vi "Teleop.vi"(10 "Match Info":T1={"Autonomous Elapsed Seconds"=0.0, "TeleOp Elapsed Seconds"=0.0, "Disabled Elapsed Seconds"=0.0, "Visited Autonomous"=FALSE, "Visited TeleOp"=FALSE, "Visited Disabled"=FALSE, "Autonomous Settings"={"Autonomous Style"=enum."Independent", "VI Refnum"=refnum}}, 11 "Call Context":T2) -> ()   [LabVIEW 2023]
doc: "This VI is called for each TeleOp packet received from the DS where the robot is not disabled. It is often used to read from the joysticks and update I/O or to update setpoints for timed control loops. It should complete and return within 20 milliseconds or it may miss DS packets."
uses:
  <vilib>/Rock Robotics/WPI/DriverStation/WPI_DriverStationDerivedRobotMode.ctl
  <vilib>/Rock Robotics/WPI/DriverStation/WPI_DriverStationMatch Info.ctl
  <vilib>/Rock Robotics/WPI/Utilities/WPI_GetSetVariantRefNum.vi
  <vilib>/Rock Robotics/Network Tables/NT Write Boolean Array.vi
  <vilib>/Rock Robotics/Network Tables/NT Write Numeric Array.vi
  <vilib>/Rock Robotics/Network Tables/NT Write Boolean.vi
  <vilib>/Rock Robotics/Network Tables/NT Read Boolean.vi
  <vilib>/Rock Robotics/Network Tables/NT Read Number.vi
  <vilib>/Rock Robotics/WPI/RobotDrive/WPI_RobotDriveMecanumDrive_Cartesian.vi
panel:
  out "Sample Slider 0":dbl(slide) scale=0.0..5.0
  out "Sample Boolean 1":bool
  out "Sample Boolean 0":bool
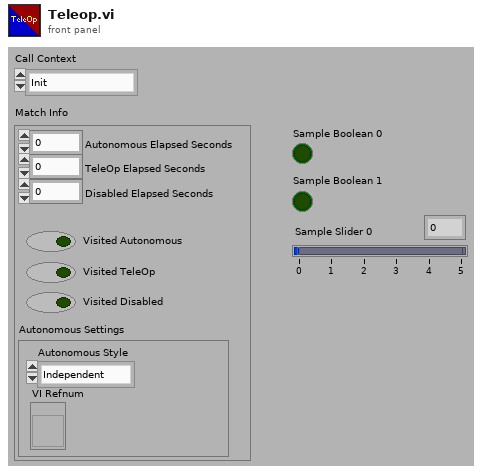
[diagram p1: front panel]
types:
  T1 = typedef "WPI_DriverStationMatch Info.ctl" = cluster{"Autonomous Elapsed Seconds":dbl, "TeleOp Elapsed Seconds":dbl, "Disabled Elapsed Seconds":dbl, "Visited Autonomous":bool, "Visited TeleOp":bool, "Visited Disabled":bool, "Autonomous Settings":cluster{"Autonomous Style":enum16{"Iterative", "Independent"}, "VI Refnum":refnum<vi>}}
  T2 = typedef "WPI_DriverStationDerivedRobotMode.ctl" = enum16{"Init", "Execute", "Stop"}
  T3 = typedef "WPI_MotorControlDeviceRef.ctl" = cluster{"DeviceStatus":errorcluster, "Type":T4, "PWM":cluster{"PWM Channel":T5, "DeadBand":T6}, "CAN":cluster{"Device Number":u8, "SetOutput VI Ref":variant, "GetOutput VI Ref":variant, "Enable VI Ref":variant, "Disable VI Ref":variant, "Data":variant}, "Invert":bool, "DIO PWM":cluster{"PWM \"Enable\" Channel":T5, "DIOChannel":T7, "PWM Rate":dbl}}
  T4 = typedef "WPI_MotorControlType.ctl" = enum16{"PWM", "CAN", "DIO PWM"}
  T5 = typedef "FPGA_DIOPWMChannel.ctl" = enum8{"PWM 0", "PWM 1", "PWM 2", "PWM 3", "PWM 4", "PWM 5", "PWM 6", "PWM 7", "PWM 8", "PWM 9", "PWM MXP 0", "PWM MXP 1", "PWM MXP 2", "PWM MXP 3", "PWM MXP 4", "PWM MXP 5", "PWM MXP 6", "PWM MXP 7", "PWM MXP 8", "PWM MXP 9", "Invalid"}
  T6 = typedef "WPI_PWMDeadband.ctl" = cluster{"Name":string, "maxPositivePwm":i32, "minPositivePwm":i32, "centerPwm":i32, "maxNegativePwm":i32, "minNegativePwm":i32, "angularRange":u16}
  T7 = typedef "FPGA_DIOChannel.ctl" = enum8{"DIO 0", "DIO 1", "DIO 2", "DIO 3", "DIO 4", "DIO 5", "DIO 6", "DIO 7", "DIO 8", "DIO 9", "DIO MXP 0", "DIO MXP 1", "DIO MXP 2", "DIO MXP 3", "DIO MXP 4", "DIO MXP 5", "DIO MXP 6", "DIO MXP 7", "DIO MXP 8", "DIO MXP 9", "DIO MXP 10", "DIO MXP 11", "DIO MXP 12", "DIO MXP 13", "DIO MXP 14", "DIO MXP 15", "SPI Port CS1", "SPI Port CS2", "SPI Port CS3", "SPI Port MISO", "SPI Port MOSI", "Invalid"}
  T8 = typedef "WPI_JoystickDevRef.ctl" = cluster{"Device":T9}
  T9 = typedef "WPI_JoystickDeviceEnum.ctl" = enum16{"USB 0", "USB 1", "USB 2", "USB 3", "USB 4", "USB 5"}
  T10 = typedef "WPI_RobotDriveDevRef.ctl" = cluster{"DevStatus":errorcluster, "Motors[]":T3[], "Square Inputs":bool, "Max Output":dbl}
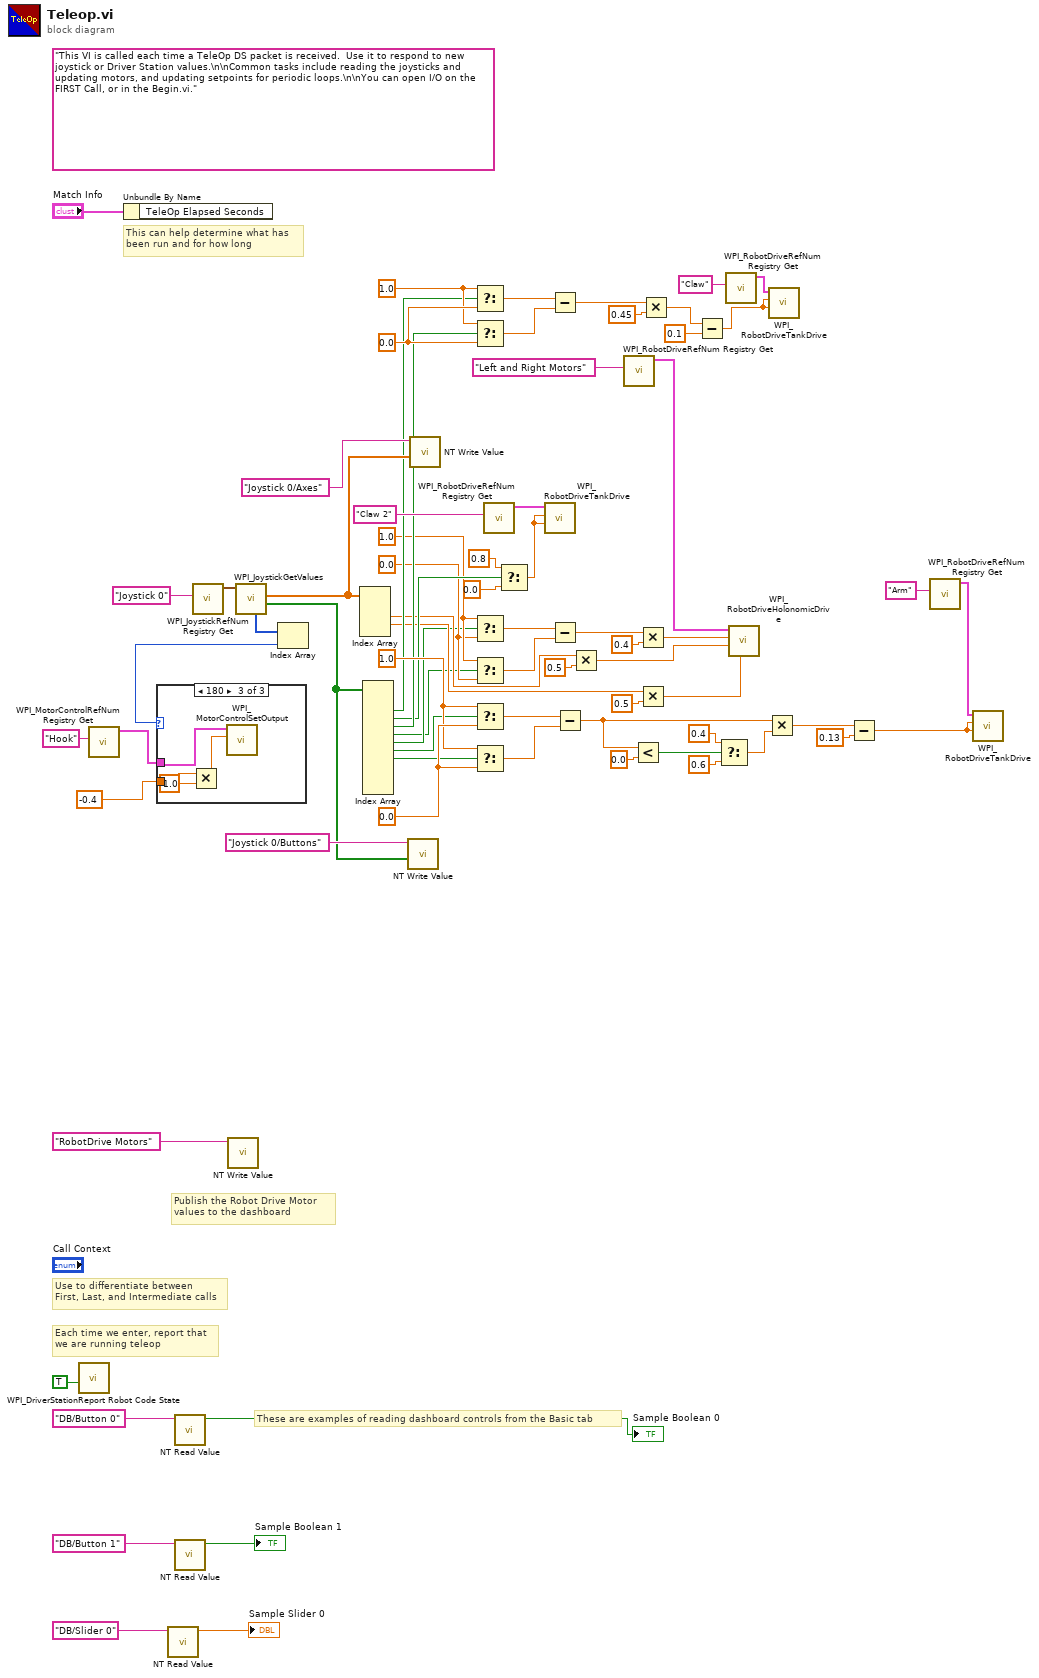
[diagram p0: block diagram]
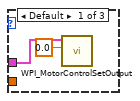
[diagram p2: hidden frame]
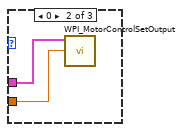
[diagram p3: hidden frame]
diagram:
  w12 = 0.0 ("f")
  w13 = 1.0 ("t")
  w42 = 1.0 ("f")
  w43 = 0.0 ("f")
  w47 = 1.0 ("f")
  w48 = 0.0 ("f")
  (unwired) "This VI is called each time a TeleOp DS packet is received.  Use it to respond to new joystick or Driver Station values.\n\nCommon tasks include reading the joysticks and updating motors, and updating setpoints for periodic loops.\n\nYou can open I/O on the FIRST Call, or in the Begin.vi."
  # "These are examples of reading dashboard controls from the Basic tab"
  # "Publish the Robot Drive Motor\nvalues to the dashboard"
  # "Each time we enter, report that\nwe are running teleop"
  # "Use to differentiate between\nFirst, Last, and Intermediate calls"
  # "This can help determine what has\nbeen run and for how long"
  n1 = call <vilib>:"WPI_DriverStationReport Robot Code State.vi"("TeleOp"=TRUE ("Autonomous")) -> ()  [unwired: 10 in, 1 out]
  n2 = call <vilib>:"WPI_MotorControlRefNum Registry Get.vi"("refnum name"="Hook") -> ("MotorControlDevRef"=w6:T3)  [unwired: 9 in, 1 out]
  n3 = Unbundle By Name("Match Info") -> ()  [unwired: 1 out]
  n4 = call-poly <vilib>:"NT Read Value.vi"("name"="DB/Slider 0" ("refnum name")) -> ("value"=→"Sample Slider 0":dbl)  [unwired: 8 in, 2 out]
  n5 = call-poly <vilib>:"NT Read Value.vi"("name"="DB/Button 0" ("refnum name")) -> ("value"=→"Sample Boolean 0":bool)  [unwired: 8 in, 2 out]
  n6 = call-poly <vilib>:"NT Read Value.vi"("name"="DB/Button 1" ("refnum name")) -> ("value"=→"Sample Boolean 1":bool)  [unwired: 8 in, 2 out]
  n7 = call <vilib>:"WPI_JoystickRefNum Registry Get.vi"("refnum name"="Joystick 0") -> ("JoystickDevRef"=w70:T8)  [unwired: 1 in, 9 out]
  n8 = call-poly <vilib>:"NT Write Value.vi"("name"="RobotDrive Motors" ("Name")) -> ()  [unwired: 10 in, 1 out]
  n9 = call <vilib>:"WPI_JoystickGetValues.vi"("JoystickDevRef"=w70) -> ("Buttons"=w49:bool[], "Axes"=w51:dbl[], "POVs"=w31:i16[])  [unwired: 6 in, 2 out]
  n10 = Index Array(array=w31) -> (element=w7:i16)  [unwired: 1 in]
  n11 = case shown="180" w7 {
    tunnel: w6 -> [w75 w77 w81]
    tunnel: -0.4 -> [_ w76 w80]
    frame Default {
      n12 = call <vilib>:"WPI_MotorControlSetOutput.vi"("Output"=0.0, "MotorControlDevRef"=w75) -> ()  [unwired: 7 in, 3 out]
    }
    frame 0 {
      n13 = call <vilib>:"WPI_MotorControlSetOutput.vi"("Output"=w76, "MotorControlDevRef"=w77) -> ()  [unwired: 7 in, 3 out]
    }
    frame 180 {
      n14 = Multiply(x=w80, y=-1.0) -> (x*y=w78:dbl)
      n15 = call <vilib>:"WPI_MotorControlSetOutput.vi"("Output"=w78, "MotorControlDevRef"=w81) -> ()  [unwired: 7 in, 3 out]
    }
  }
  n16 = Index Array(array=w51) -> (element #2=w25:dbl, element #3=w24:dbl)  [unwired: 4 in, 2 out]
  n17 = Index Array(array=w49) -> (element #2=w30:bool, element #3=w26:bool, element #4=w27:bool, element #5=w8:bool, element #6=w11:bool, element #7=w10:bool, element #8=w16:bool)  [unwired: 12 in, 5 out]
  n18 = call-poly <vilib>:"NT Write Value.vi"("value"=w49, "name"="Joystick 0/Buttons" ("Name")) -> ()  [unwired: 9 in, 1 out]
  n19 = call-poly <vilib>:"NT Write Value.vi"("value"=w51, "name"="Joystick 0/Axes" ("Name")) -> ()  [unwired: 9 in, 1 out]
  n20 = Select(t=w47, s=w30, f=w48) -> (s? t:f=w46:dbl)
  n21 = Select(t=w47, s=w27, f=w48) -> (s? t:f=w45:dbl)
  n22 = Select(t=w13, s=w11, f=w12) -> (s? t:f=w14:dbl)
  n23 = Select(t=w13, s=w8, f=w12) -> (s? t:f=w15:dbl)
  n24 = Select(t=w42, s=w10, f=w43) -> (s? t:f=w40:dbl)
  n25 = Select(t=w42, s=w16, f=w43) -> (s? t:f=w41:dbl)
  n26 = call <vilib>:"WPI_RobotDriveRefNum Registry Get.vi"("refnum name"="Claw 2") -> ("RobotDriveDevRef"=w39:T10)  [unwired: 1 in, 9 out]
  n27 = Select(t=0.8, s=w26, f=0.0) -> (s? t:f=w37:dbl)
  n28 = call <vilib>:"WPI_RobotDriveTankDrive.vi"("Right axis value"=w37, "Left axis value"=w37, "RobotDriveDevRef"=w39) -> ()  [unwired: 6 in, 3 out]
  n29 = Subtract(x=w46, y=w45) -> (x-y=w32:dbl)
  n30 = Subtract(x=w14, y=w15) -> (x-y=w9:dbl)
  n31 = Subtract(x=w40, y=w41) -> (x-y=w22:dbl)
  n32 = Multiply(x=w25, y=0.5) -> (x*y=w54:dbl)
  n33 = call <vilib>:"WPI_RobotDriveRefNum Registry Get.vi"("refnum name"="Left and Right Motors") -> ("RobotDriveDevRef"=w59:T10)  [unwired: 1 in, 9 out]
  n34 = Less?(x=w22, y=0.0) -> (x < y?=w20:bool)
  n35 = Multiply(x=w9, y=0.4) -> (x*y=w55:dbl)
  n36 = Multiply(x=w24, y=0.5) -> (x*y=w53:dbl)
  n37 = Multiply(x=w32, y=0.45 ("x")) -> (x*y=w2:dbl)
  n38 = Subtract(x=w2, y=0.1) -> (x-y=w1:dbl)
  n39 = Select(t=0.4, s=w20, f=0.6) -> (s? t:f=w17:dbl)
  n40 = call <vilib>:"WPI_RobotDriveRefNum Registry Get.vi"("refnum name"="Claw") -> ("RobotDriveDevRef"=w50:T10)  [unwired: 1 in, 9 out]
  n41 = call-poly <vilib>:"WPI_RobotDriveHolonomicDrive.vi"("Rotation"=w53, "Y"=w54, "X"=w55, "RobotDriveDevRef"=w59) -> ()  [unwired: 5 in, 3 out]
  n42 = Multiply(x=w22, y=w17) -> (x*y=w23:dbl)
  n43 = call <vilib>:"WPI_RobotDriveTankDrive.vi"("Right axis value"=w1, "Left axis value"=w1, "RobotDriveDevRef"=w50) -> ()  [unwired: 6 in, 3 out]
  n44 = Subtract(x=w23, y=0.13) -> (x-y=w33:dbl)
  n45 = call <vilib>:"WPI_RobotDriveRefNum Registry Get.vi"("refnum name"="Arm") -> ("RobotDriveDevRef"=w29:T10)  [unwired: 1 in, 9 out]
  n46 = call <vilib>:"WPI_RobotDriveTankDrive.vi"("Right axis value"=w33, "Left axis value"=w33, "RobotDriveDevRef"=w29) -> ()  [unwired: 6 in, 3 out]
